vi "seqPrg.vi"() -> ()   [LabVIEW 2019]
panel:
  out "CopyVISAsession":refnum<visa-resource-name>
  in  "Tab Control":enum32{"Manual", "SEQ"}(tab)
  in  "read":bool
  in  "output":bool
  in  "Operation mode":u16(ring) items=["CV-INT", "CV-EXT", "CV-ADD", "CC-INT", "CC-EXT", "CC-ADD"]
  in  "Current[A]":dbl(knob) min=-20.0 max=20.0 step=0.001 scale=-20.0..20.0
  in  "Current[Ap-p]":dbl(knob) min=0.0 max=60.0 step=0.01 scale=0.0..60.0
  in  "Voltage[Vp-p]":dbl(knob) min=0.0 max=120.0 step=0.1 scale=0.0..120.0
  in  "Voltage[V]":dbl(knob) min=-115.0 max=115.0 step=0.01 scale=-115.0..115.0
  in  "Waveform":u16(ring) items=["Sine", "Square", "ARB 1", "ARB 2", "ARB 3", "ARB 4", "ARB 5", "ARB 6", "ARB 7", "ARB 8", "ARB 9", "ARB 10", "ARB 11", "ARB 12", "ARB 13", "ARB 14", "ARB 15", "ARB 16"]
  in  "Frequency[Hz]":dbl(knob)=1.0 min=1.0 max=100000.0 step=0.1 scale=1.0..100000.0
  in  "Set":enum16{"Current", "Voltage", "FREQ/WAVE"}(ring)=enum."Voltage"
  out "AC current[Ap-p]":dbl format="%.1f"
  out "AC voltage[Vp-p]":dbl
  out "DC current[A]":dbl format="%.2f"
  out "DC voltage[V]":dbl format="%.1f"
  in  "seq_scjn":bool
  out "Query":i32
  out "Read Data txt":string
  in  "seq_scsn":bool
  in  "seq_sctl":bool
  in  "Controls the sequence":u32(ring) items=["STOP", "START", "HOLD", "BRANCH1", "BRANCH2"]
  in  "seq_seqm":bool
  in  "seq_sexp":bool
  in  "Parameter":T1={"1st"=0.0, "2nd"=0, "3rd"=0.0, "4th"=0, "5th"=1.0, "6th"=0, "7th"=2, "8th"=0, "9th"=0, "10th"=0} {"10th" items=["CONST", "KEEP"]; "9th" items=["(0,0)", "(0,1)", "(1,0)", "(1,1)"]; "8th" items=["CONST", "KEEP"]; "7th" items=["ARB 1"=2, "ARB 2"=3, "ARB 3"=4, "ARB 4"=5, "ARB 5"=6, "ARB 6"=7, "ARB 7"=8, "ARB 8"=9, "ARB 9"=10, "ARB 10"=11, "ARB 11"=12, "ARB 12"=13, "ARB 13"=14, "ARB 14"=15, "ARB 15"=16, "ARB 16"=17]; "6th" items=["CONST", "KEEP", "SWEEP"]; "5th" min=1.0 max=100000.0 step=0.1 format="%.1f"; "4th" items=["CONST", "KEEP", "SWEEP"]; "3rd" min=0.0 max=120.0 step=0.01 format="%.2f"; "2nd" items=["CONST", "KEEP", "SWEEP"]; "1st" min=-115.0 max=115.0 step=0.001 format="%.3f"}
  in  "seq_slen":bool
  in  "seq_ssts":bool
  in  "seq_stpn":bool
  in  "STEP":dbl=1.0 min=1.0 max=255.0 step=1.0
  out "Query 2":dbl=999.0 caption="Query"
  out "Read Data txt 2":string caption="Read Data txt"
  in  "seq_strp":bool
  in  "Parameter 2":T2={"1st"=0, "2nd"=0.1, "3rd"=0, "4th"=0, "5th"=0, "6th"=1, "7th"=1, "8th"=1, "9th"=1} caption="Parameter" {"9th" min=0 max=255 step=1; "8th" min=0 max=255 step=1; "7th" min=0 max=999 step=1; "6th" min=0 max=255 step=1; "5th" items=["CONTINUE", "IDLE", "HOLD"]; "4th" min=0 max=0; "3rd" items=["DISABLE", "ENABLE"]; "2nd" min=0.0001 max=999.9999 step=0.0001 format="%.4f"; "1st" min=0 max=0}
  out "Query 3":string caption="Query"
  out "Query 4":string caption="Query"
  in  "Read(F)":bool
  in  "Read(F) 2":bool caption="Read(F)"
  in  "Read(F) 3":bool caption="Read(F)"
  in  "close":bool
  in  "open":bool
  in  "VISAsession":refnum<visa-resource-name>
  in  "stop":bool
  # "세팅순서\n\nseq_strp 세팅: 시간\nseq_seqm 세팅: 레벨\nseq_slen 세팅: 스텝\nseq_sctl: 시퀀스 시작"
  # "fixed"
  # "fixed"
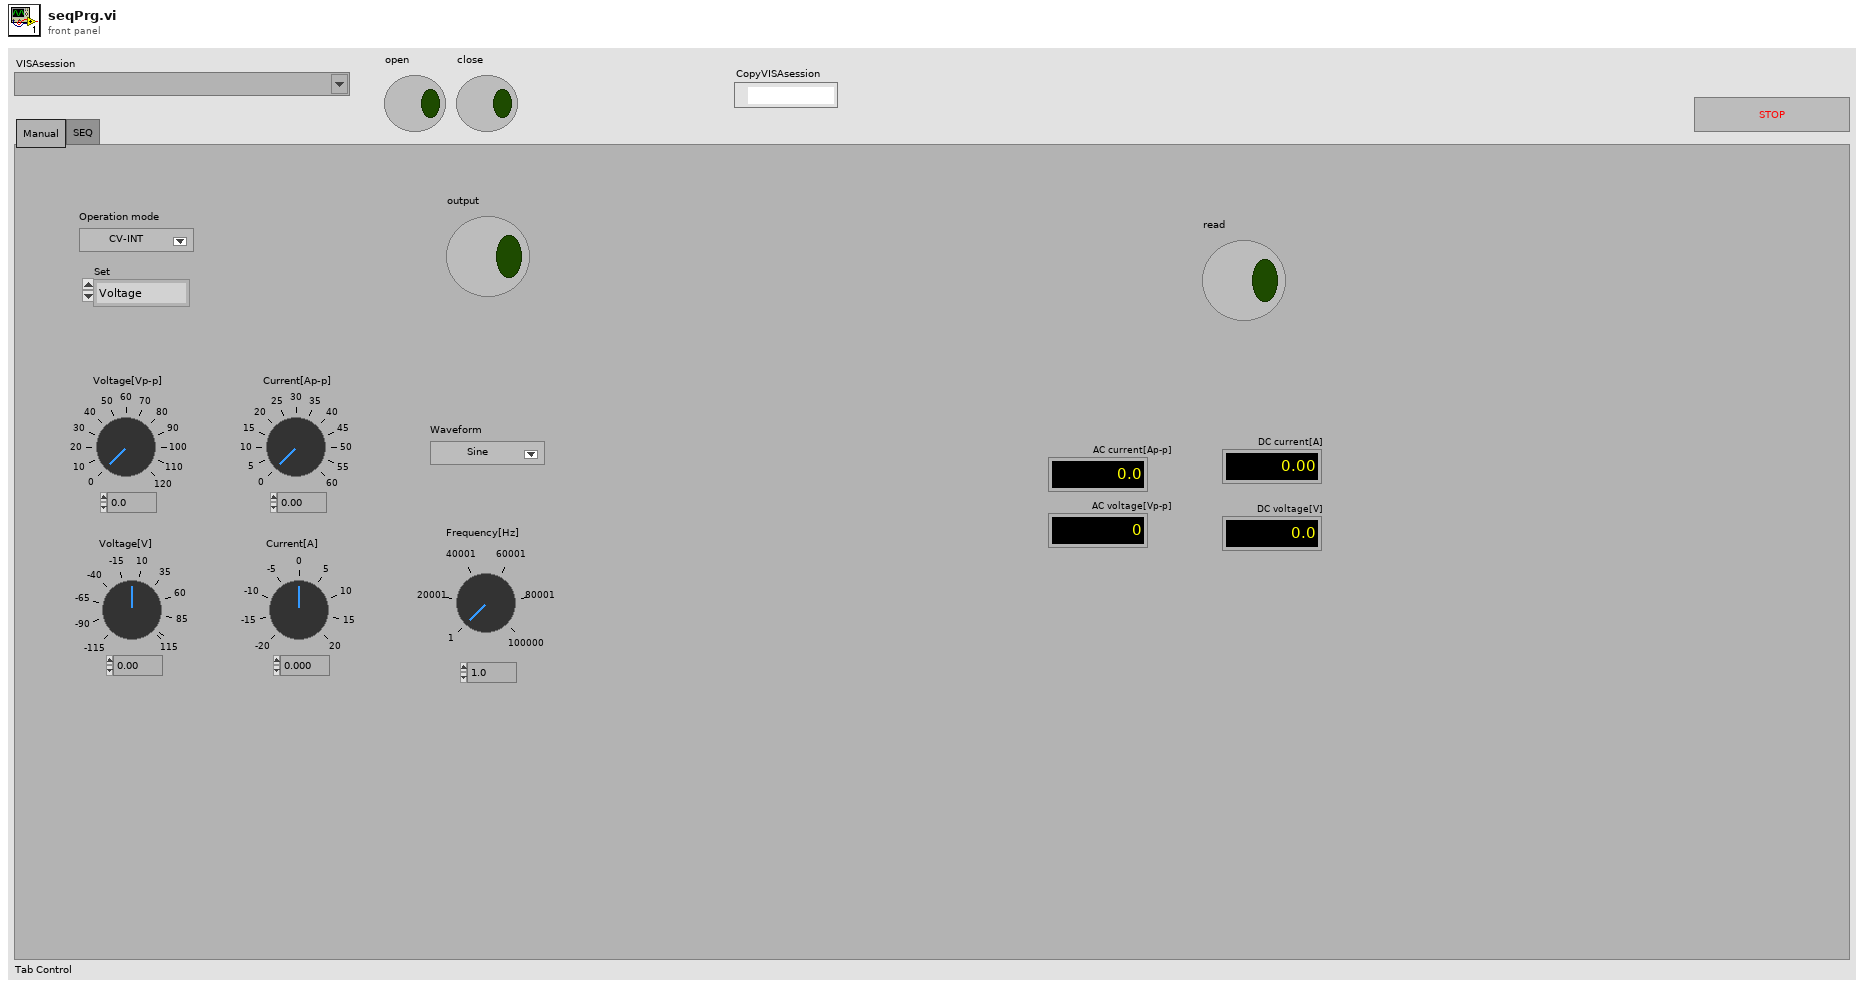
[diagram p1: front panel]
types:
  T1 = cluster{"1st":dbl, "2nd":u16, "3rd":dbl, "4th":u16, "5th":dbl, "6th":u16, "7th":u16, "8th":u16, "9th":u16, "10th":u16}
  T2 = cluster{"1st":i8, "2nd":dbl, "3rd":u16, "4th":i8, "5th":u16, "6th":i32, "7th":i32, "8th":i32, "9th":i32}
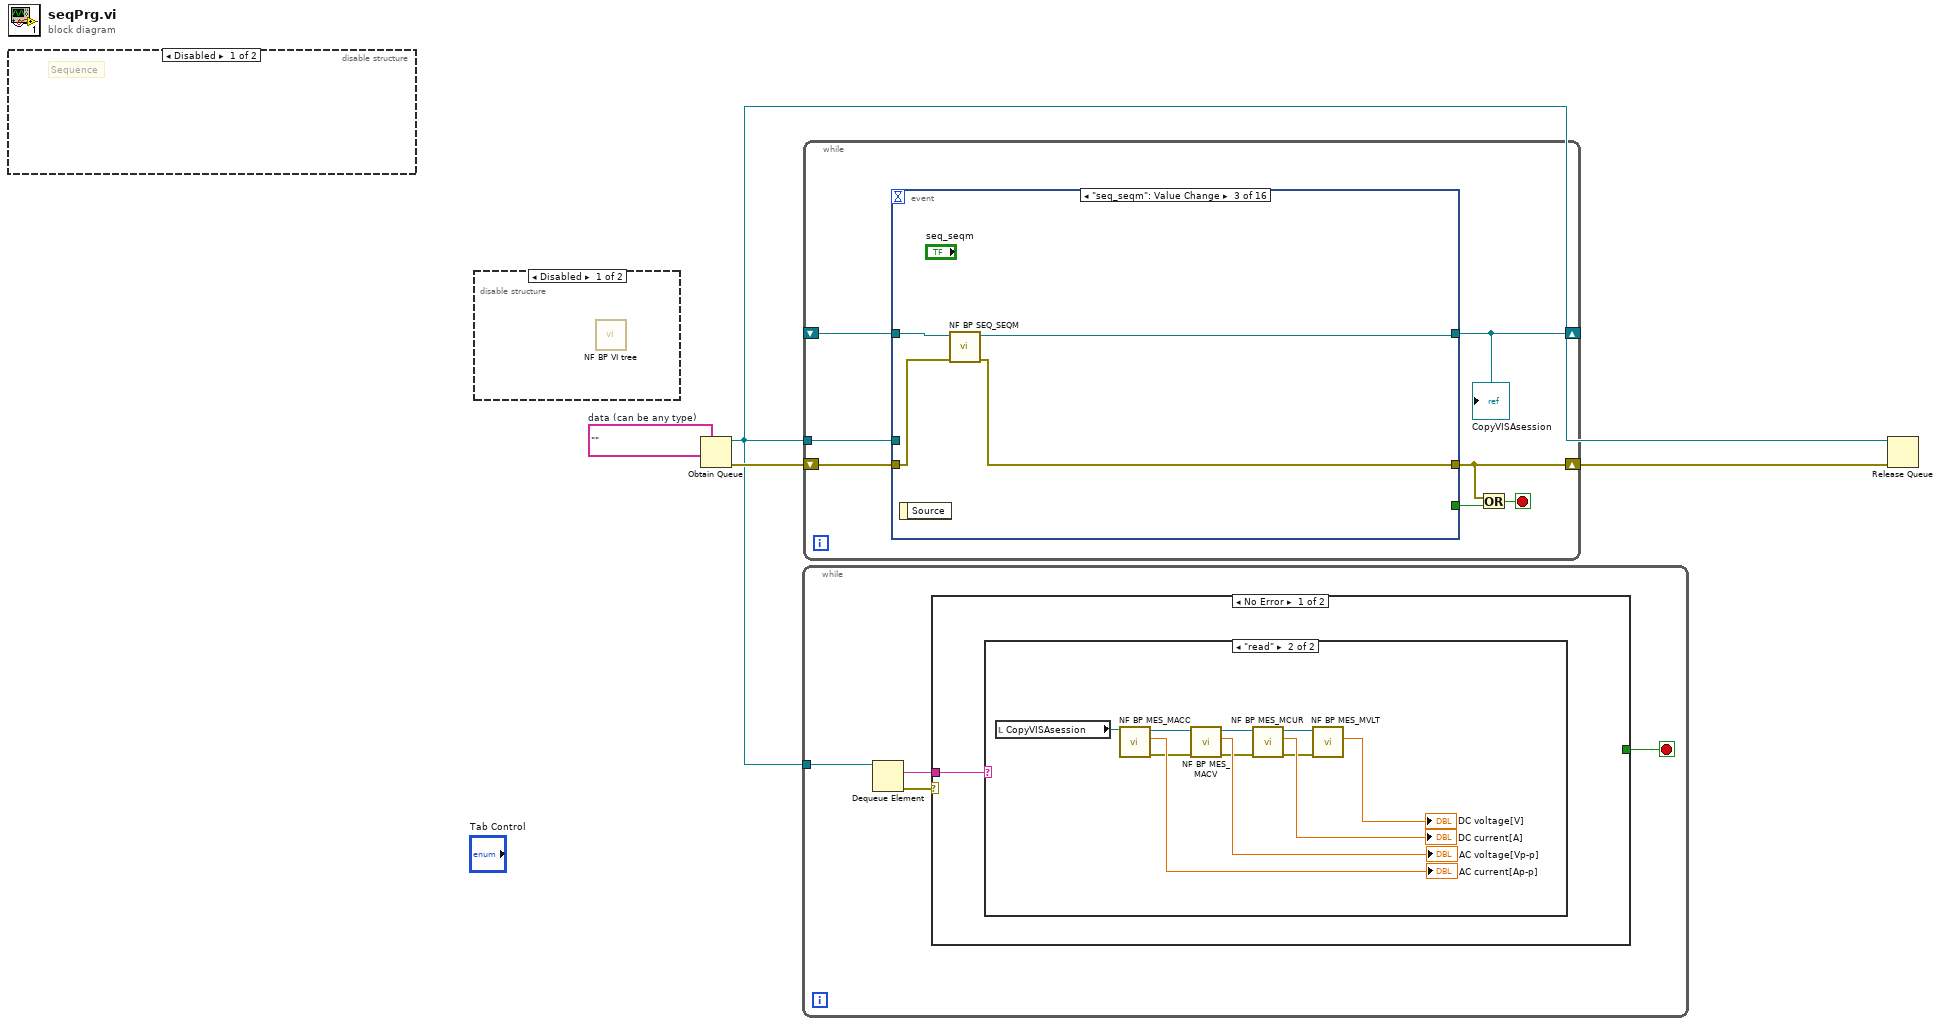
[diagram p0: block diagram]
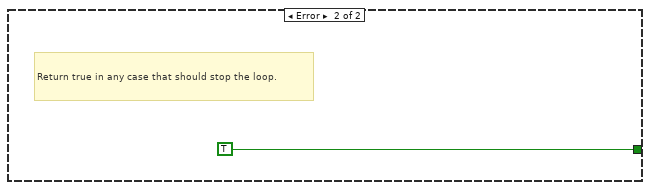
[diagram p5: hidden frame]
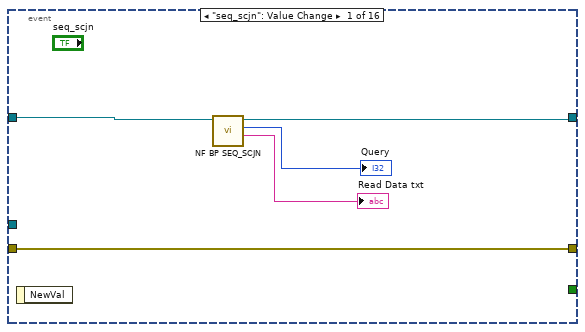
[diagram p6: hidden frame]
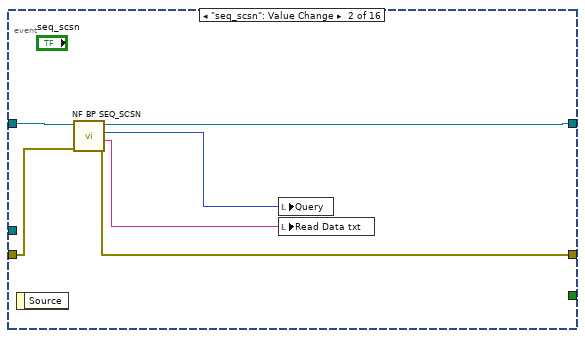
[diagram p7: hidden frame]
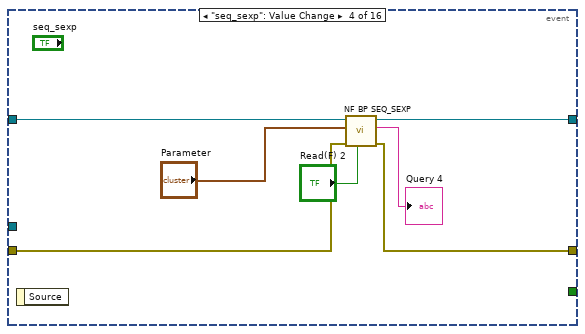
[diagram p8: hidden frame]
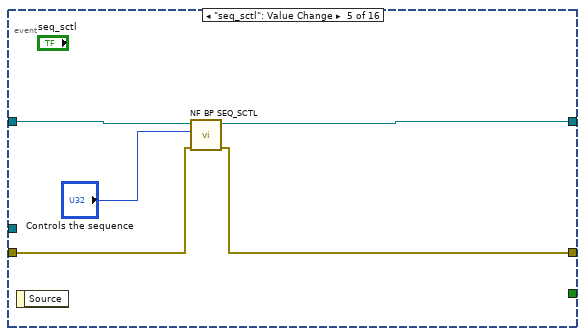
[diagram p9: hidden frame]
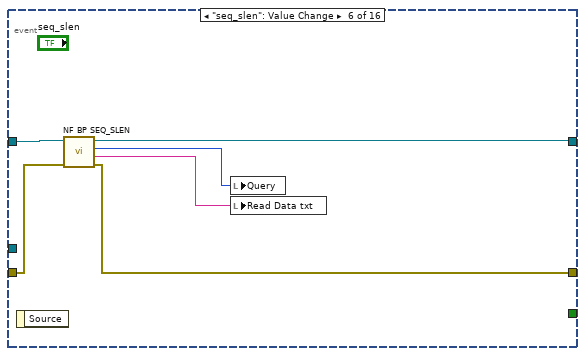
[diagram p10: hidden frame]
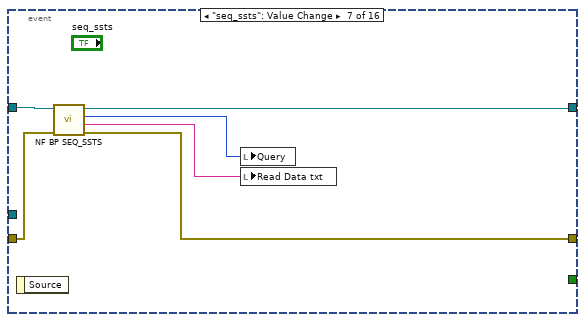
[diagram p11: hidden frame]
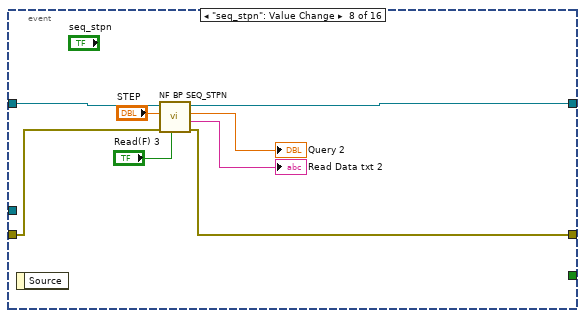
[diagram p12: hidden frame]
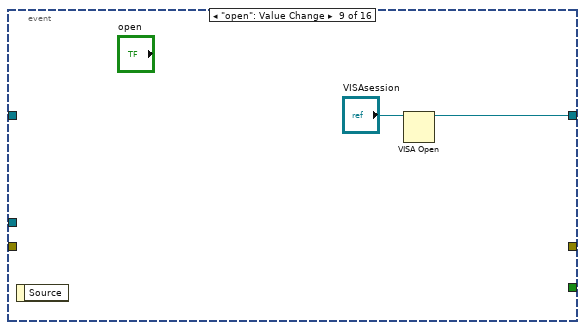
[diagram p13: hidden frame]
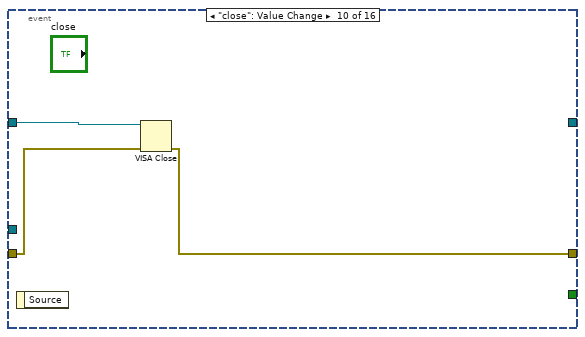
[diagram p14: hidden frame]
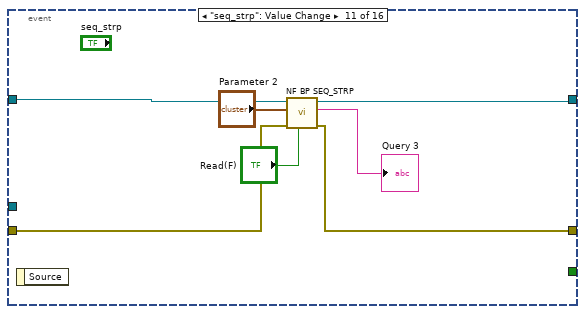
[diagram p15: hidden frame]
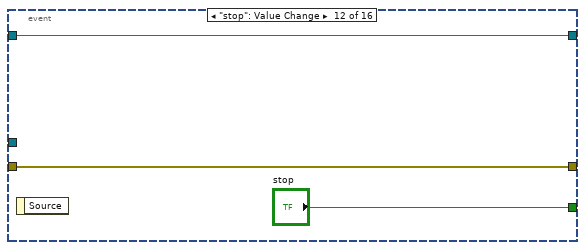
[diagram p16: hidden frame]
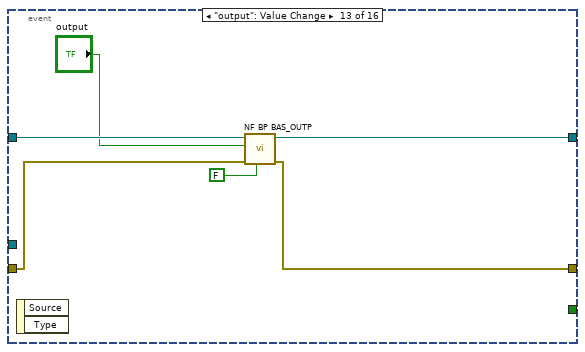
[diagram p17: hidden frame]
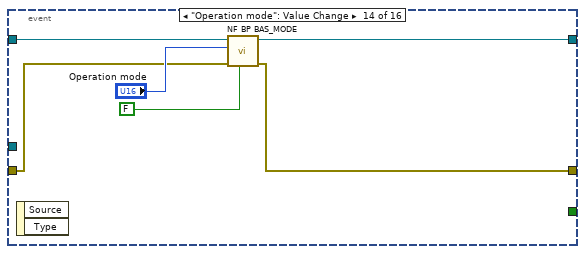
[diagram p18: hidden frame]
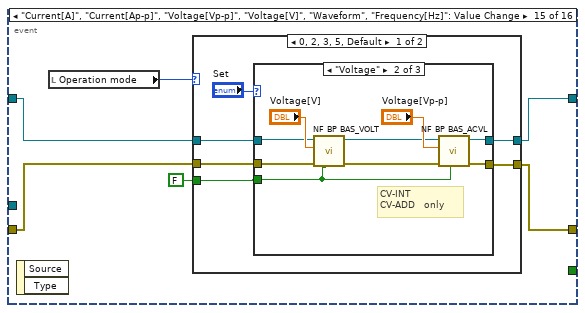
[diagram p19: hidden frame]
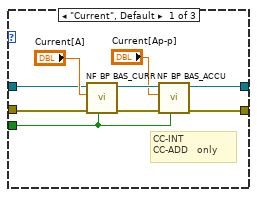
[diagram p20: hidden frame]
diagram:
  w2 = ""  # data (can be any type)
  n1 = disable-structure shown="Disabled" {
    frame Disabled {
      # "Sequence"
    }
    frame Enabled {
    }
  }
  n2 = disable-structure shown="Disabled" {
    frame Disabled {
      n3 = call <instrlib>:"NF BP VI tree.vi"() -> ()  [unwired: 1 in]
    }
    frame Enabled {
    }
  }
  n4 = Obtain Queue(element data type=w2) -> (queue out=w1:refnum<queue>, error out=w4:errorcluster)  [unwired: 4 in, 1 out]
  n5 = while {
    tunnel: w1 -> [w8]
    stop <- w5 stop-if-true
    n6 = Dequeue Element(queue=w8) -> (element=w6:string, error out=w7:errorcluster)  [unwired: 2 in, 2 out]
    n7 = case shown="No Error" w7 {
      tunnel: w6 -> [w9 _]
      tunnel: [_ TRUE] -> w5
      frame No Error {
        n8 = case shown="\"read\"" w9 {
          frame "False", Default {
          }
          frame "read" {
            n9 = local read "CopyVISAsession"() -> (w10:refnum<visa-resource-name>)
            n10 = call <instrlib>:"NF BP MES_MACC.vi"("VISAsession"=w10) -> ("error out"=w11:errorcluster, "Query[Ap-p]"=→"AC current[Ap-p]":dbl, "CopyVISAsession"=w18:refnum<visa-resource-name>)  [unwired: 6 in, 2 out]
            n11 = call <instrlib>:"NF BP MES_MACV.vi"("error in (no error)"=w11, "VISAsession"=w18) -> ("error out"=w12:errorcluster, "Query[Vp-p]"=→"AC voltage[Vp-p]":dbl, "CopyVISAsession"=w19:refnum<visa-resource-name>)  [unwired: 5 in, 2 out]
            n12 = call <instrlib>:"NF BP MES_MCUR.vi"("error in (no error)"=w12, "VISAsession"=w19) -> ("error out"=w13:errorcluster, "Query[A]"=→"DC current[A]":dbl, "CopyVISAsession"=w20:refnum<visa-resource-name>)  [unwired: 5 in, 2 out]
            n13 = call <instrlib>:"NF BP MES_MVLT.vi"("error in (no error)"=w13, "VISAsession"=w20) -> ("Query[V]"=→"DC voltage[V]":dbl)  [unwired: 5 in, 4 out]
          }
        }
      }
      frame Error {
        # "Return true in any case that should stop the loop."
      }
    }
  }
  n14 = while {
    shift-right: [w24] -> w3
    shift-left: w4 -> [w27]
    tunnel: w1 -> [w28]
    shift-right: [w23] -> _
    shift-left: _ -> [w22]
    stop <- w25 stop-if-true
    n15 = event shown="[2] \"seq_seqm\": Value Change" {
      selector: _ -> [_ _ _ _ _ _ _ _ _ _ _ _ _ _ _ _]
      dyn-events: _ -> [_ _ _ _ _ _ _ _ _ _ _ _ _ _ _ _]
      timeout: _ -> [_ _ _ _ _ _ _ _ _ _ _ _ _ _ _ _]
      tunnel: w28 -> [_ _ _ _ _ _ _ _ _ _ _ _ _ _ _ w147]
      tunnel: w27 -> [w29 w35 w41 w47 w52 w57 w63 w70 _ w79 w84 w89 w93 w99 w105 w146]
      tunnel: [w29 w34 w40 w46 w51 w56 w62 w69 _ w78 w83 w89 w91 w97 w103 w145] -> w24
      tunnel: [_ _ _ _ _ _ _ _ _ _ _ "stop" _ _ _ _] -> w26
      tunnel: w22 -> [w33 w39 w43 w50 w55 w61 w67 w75 _ w80 w87 w88 w95 w100 w107 w144]
      tunnel: [w30 w36 w42 w44 w53 w58 w64 w71 w76 _ w82 w88 w94 w98 w106 w144] -> w23
      event "seq_scjn": Value Change {
        n16 = event-data() -> ()  [unwired: 1 in, 1 out]
        n17 = call <instrlib>:"NF BP SEQ_SCJN.vi"("VISAsession"=w33) -> ("Read Data txt"=→"Read Data txt":string, "Query"=→"Query":i32, "CopyVISAsession"=w30:refnum<visa-resource-name>)  [unwired: 7 in, 1 out]
      }
      event "seq_scsn": Value Change {
        n18 = event-data() -> ()  [unwired: 1 in, 1 out]
        n19 = call <instrlib>:"NF BP SEQ_SCSN.vi"("error in (no error)"=w35, "VISAsession"=w39) -> ("error out"=w34:errorcluster, "Read Data txt"=w37:string, "Query"=w38:i32, "CopyVISAsession"=w36:refnum<visa-resource-name>)  [unwired: 6 in]
        n20 = local write "Query"(w38) -> ()
        n21 = local write "Read Data txt"(w37) -> ()
      }
      event "seq_seqm": Value Change {
        n22 = event-data() -> ()  [unwired: 1 in, 1 out]
        n23 = call <instrlib>:"NF BP SEQ_SEQM.vi"("error in (no error)"=w41, "VISAsession"=w43) -> ("error out"=w40:errorcluster, "CopyVISAsession"=w42:refnum<visa-resource-name>)  [unwired: 8 in]
      }
      event "seq_sexp": Value Change {
        n24 = event-data() -> ()  [unwired: 1 in, 1 out]
        n25 = call <instrlib>:"NF BP SEQ_SEXP.vi"("Read(F)"="Read(F) 2", "error in (no error)"=w47, "Parameter"="Parameter", "VISAsession"=w50) -> ("error out"=w46:errorcluster, "Query"=→"Query 4":string, "CopyVISAsession"=w44:refnum<visa-resource-name>)  [unwired: 5 in]
      }
      event "seq_sctl": Value Change {
        n26 = event-data() -> ()  [unwired: 1 in, 1 out]
        n27 = call <instrlib>:"NF BP SEQ_SCTL.vi"("error in (no error)"=w52, "Controls the sequence"="Controls the sequence", "VISAsession"=w55) -> ("error out"=w51:errorcluster, "CopyVISAsession"=w53:refnum<visa-resource-name>)  [unwired: 7 in]
      }
      event "seq_slen": Value Change {
        n28 = event-data() -> ()  [unwired: 1 in, 1 out]
        n29 = call <instrlib>:"NF BP SEQ_SLEN.vi"("error in (no error)"=w57, "VISAsession"=w61) -> ("error out"=w56:errorcluster, "Read Data txt"=w59:string, "Query"=w60:i32, "CopyVISAsession"=w58:refnum<visa-resource-name>)  [unwired: 6 in]
        n30 = local write "Query"(w60) -> ()
        n31 = local write "Read Data txt"(w59) -> ()
      }
      event "seq_ssts": Value Change {
        n32 = event-data() -> ()  [unwired: 1 in, 1 out]
        n33 = call <instrlib>:"NF BP SEQ_SSTS.vi"("error in (no error)"=w63, "VISAsession"=w67) -> ("error out"=w62:errorcluster, "Read Data txt"=w65:string, "Query"=w66:i32, "CopyVISAsession"=w64:refnum<visa-resource-name>)  [unwired: 6 in]
        n34 = local write "Query"(w66) -> ()
        n35 = local write "Read Data txt"(w65) -> ()
      }
      event "seq_stpn": Value Change {
        n36 = event-data() -> ()  [unwired: 1 in, 1 out]
        n37 = call <instrlib>:"NF BP SEQ_STPN.vi"("Read(F)"="Read(F) 3", "error in (no error)"=w70, "STEP"="STEP", "VISAsession"=w75) -> ("error out"=w69:errorcluster, "Read Data txt"=→"Read Data txt 2":string, "Query"=→"Query 2":dbl, "CopyVISAsession"=w71:refnum<visa-resource-name>)  [unwired: 4 in]
      }
      event "open": Value Change {
        n38 = event-data() -> ()  [unwired: 1 in, 1 out]
        n39 = VISA Open(VISA resource name="VISAsession") -> (VISA resource name=w76:refnum<visa-resource-name>)  [unwired: 4 in, 1 out]
      }
      event "close": Value Change {
        n40 = event-data() -> ()  [unwired: 1 in, 1 out]
        n41 = VISA Close(VISA resource name=w80, error in (no error)=w79) -> (error out=w78:errorcluster)
      }
      event "seq_strp": Value Change {
        n42 = event-data() -> ()  [unwired: 1 in, 1 out]
        n43 = call <instrlib>:"NF BP SEQ_STRP.vi"("Read(F)"="Read(F)", "error in (no error)"=w84, "Parameter"="Parameter 2", "VISAsession"=w87) -> ("error out"=w83:errorcluster, "Query"=→"Query 3":string, "CopyVISAsession"=w82:refnum<visa-resource-name>)  [unwired: 5 in]
      }
      event "stop": Value Change {
        n44 = event-data() -> ()  [unwired: 1 in, 1 out]
      }
      event "output": Value Change {
        n45 = event-data() -> ()  [unwired: 1 in, 2 out]
        n46 = call <instrlib>:"NF BP BAS_OUTP.vi"("Read(F)"=FALSE ("Read"), "error in (no error)"=w93, "State(OFF)"="output", "VISAsession"=w95) -> ("error out"=w91:errorcluster, "CopyVISAsession"=w94:refnum<visa-resource-name>)  [unwired: 4 in, 2 out]
      }
      event "Operation mode": Value Change {
        n47 = event-data() -> ()  [unwired: 1 in, 2 out]
        n48 = call <instrlib>:"NF BP BAS_MODE.vi"("Read(F)"=FALSE ("Read"), "error in (no error)"=w99, "Select Mode"="Operation mode", "VISAsession"=w100) -> ("error out"=w97:errorcluster, "CopyVISAsession"=w98:refnum<visa-resource-name>)  [unwired: 4 in, 2 out]
      }
      event "Current[A]", "Current[Ap-p]", "Voltage[Vp-p]", "Voltage[V]", "Waveform", "Frequency[Hz]": Value Change {
        n49 = event-data() -> ()  [unwired: 1 in, 2 out]
        n50 = local read "Operation mode"() -> (w108:u16)
        n51 = case shown="0, 2, 3, 5, Default" w108 {
          tunnel: w107 -> [w113 w143]
          tunnel: w105 -> [w112 w142]
          tunnel: [w111 w143] -> w106
          tunnel: [w110 w142] -> w103
          tunnel: FALSE ("Read") -> [w109 _]
          frame 0, 2, 3, 5, Default {
            n52 = case shown="\"Voltage\"" "Set" {
              tunnel: w112 -> [w120 w131 w141]
              tunnel: w113 -> [w118 w126 w136]
              tunnel: [w123 w128 w137] -> w110
              tunnel: w109 -> [w119 w127 w138]
              tunnel: [w115 w124 w134] -> w111
              frame "Current", Default {
                # "CC-INT\nCC-ADD   only"
                n53 = call <instrlib>:"NF BP BAS_CURR.vi"("Read(F)"=w119, "error in (no error)"=w120, "Current[A]"="Current[A]", "VISAsession"=w118) -> ("error out"=w121:errorcluster, "CopyVISAsession"=w117:refnum<visa-resource-name>)  [unwired: 4 in, 2 out]
                n54 = call <instrlib>:"NF BP BAS_ACCU.vi"("Read(F)"=w119, "error in (no error)"=w121, "Current[Ap-p]"="Current[Ap-p]", "VISAsession"=w117) -> ("error out"=w123:errorcluster, "CopyVISAsession"=w115:refnum<visa-resource-name>)  [unwired: 4 in, 2 out]
              }
              frame "Voltage" {
                # "CV-INT\nCV-ADD   only"
                n55 = call <instrlib>:"NF BP BAS_VOLT.vi"("Read(F)"=w127, "error in (no error)"=w131, "Voltage[V]"="Voltage[V]", "VISAsession"=w126) -> ("error out"=w129:errorcluster, "CopyVISAsession"=w125:refnum<visa-resource-name>)  [unwired: 4 in, 2 out]
                n56 = call <instrlib>:"NF BP BAS_ACVL.vi"("Read(F)"=w127, "error in (no error)"=w129, "Voltage[Vp-p]"="Voltage[Vp-p]", "VISAsession"=w125) -> ("error out"=w128:errorcluster, "CopyVISAsession"=w124:refnum<visa-resource-name>)  [unwired: 4 in, 2 out]
              }
              frame "FREQ/WAVE" {
                n57 = call <instrlib>:"NF BP BAS_FREQ.vi"("Read(F)"=w138, "error in (no error)"=w141, "Frequency[Hz]"="Frequency[Hz]", "VISAsession"=w136) -> ("error out"=w139:errorcluster, "CopyVISAsession"=w135:refnum<visa-resource-name>)  [unwired: 4 in, 2 out]
                n58 = call <instrlib>:"NF BP BAS_WAVE.vi"("Read(F)"=w138, "error in (no error)"=w139, "Select Function"="Waveform", "VISAsession"=w135) -> ("error out"=w137:errorcluster, "CopyVISAsession"=w134:refnum<visa-resource-name>)  [unwired: 4 in, 2 out]
              }
            }
          }
          frame 1, 4 {
          }
        }
      }
      event "read": Value Change {
        n59 = event-data() -> ()  [unwired: 1 in, 2 out]
        n60 = Enqueue Element(queue=w147, element="read", error in (no error)=w146) -> (error out=w145:errorcluster)  [unwired: 1 in, 2 out]
      }
    }
    "CopyVISAsession" <- w23
    n61 = Or(x=w24, y=w26) -> (x .or. y?=w25:bool)
  }
  n62 = Release Queue(queue=w1, error in (no error)=w3) -> ()  [unwired: 1 in, 3 out]
